vi "Actividad 1-Tanque.vi"() -> ()   [LabVIEW 2018]
panel:
  in  "stop":bool
  in  "Decremento":bool
  in  "Incremento":bool
  out "Tank":dbl(slide) scale=0.0..10.0
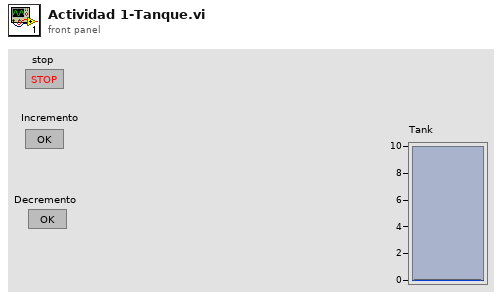
[diagram p1: front panel]
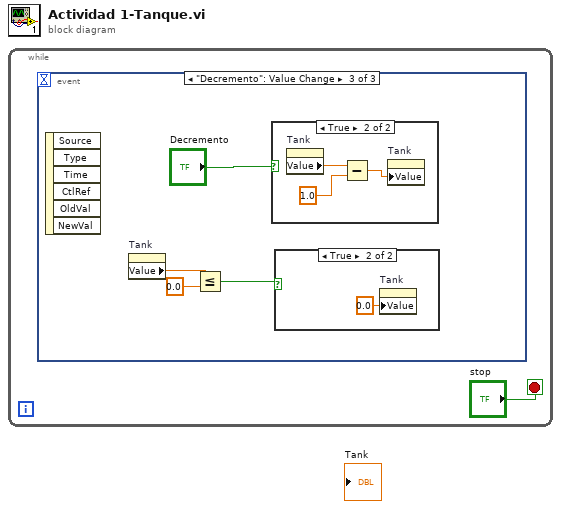
[diagram p0: block diagram]
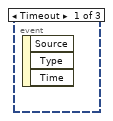
[diagram p2: hidden frame]
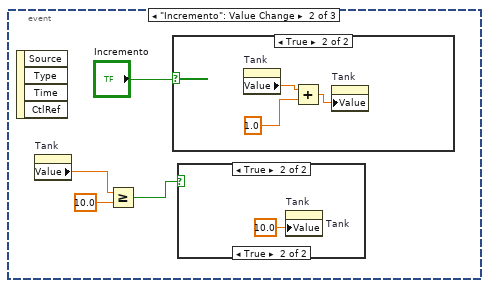
[diagram p3: hidden frame]
diagram:
  n1 = while {
    stop <- "stop" stop-if-true
    n2 = event shown="[2] \"Decremento\": Value Change" {
      selector: _ -> [_ _ _]
      dyn-events: _ -> [_ _ _]
      timeout: _ -> [_ _ _]
      event Timeout {
        n3 = event-data() -> ()  [unwired: 1 in, 3 out]
      }
      event "Incremento": Value Change {
        n4 = event-data() -> ()  [unwired: 1 in, 4 out]
        n5 = property on="Tank" class="Slide (strict)"() -> ("Value"=w3:dbl)  [unwired: 2 in, 2 out]
        n6 = Greater Or Equal?(x=w3, y=10.0) -> (x >= y?=w2:bool)
        n7 = case shown="True" "Incremento" {
          frame False {
          }
          frame True {
            n8 = property on="Tank" class="Slide (strict)"() -> ("Value"=w9:dbl)  [unwired: 2 in, 2 out]
            n9 = Add(x=w9, y=1.0) -> (x+y=w8:dbl)
            n10 = property on="Tank" class="Slide (strict)"("Value"=w8) -> ()  [unwired: 2 in, 2 out]
          }
        }
        n11 = case shown="True" {
          selector: _ -> [_ _]
          frame False {
          }
          frame True {
            n12 = property on="Tank" class="Slide (strict)"("Value"=10.0 ("Tank")) -> ()  [unwired: 2 in, 2 out]
          }
        }
        n13 = case shown="True" w2 {
          frame False {
          }
          frame True {
            n14 = property on="Tank" class="Slide (strict)"("Value"=10.0 ("Tank")) -> ()  [unwired: 2 in, 2 out]
          }
        }
      }
      event "Decremento": Value Change {
        n15 = event-data() -> ()  [unwired: 1 in, 6 out]
        n16 = property on="Tank" class="Slide (strict)"() -> ("Value"=w12:dbl)  [unwired: 2 in, 2 out]
        n17 = Less Or Equal?(x=w12, y=0.0) -> (x <= y?=w11:bool)
        n18 = case shown="True" "Decremento" {
          frame False {
          }
          frame True {
            n19 = property on="Tank" class="Slide (strict)"() -> ("Value"=w17:dbl)  [unwired: 2 in, 2 out]
            n20 = Subtract(x=w17, y=1.0) -> (x-y=w16:dbl)
            n21 = property on="Tank" class="Slide (strict)"("Value"=w16) -> ()  [unwired: 2 in, 2 out]
          }
        }
        n22 = case shown="True" w11 {
          frame False {
          }
          frame True {
            n23 = property on="Tank" class="Slide (strict)"("Value"=0.0 ("Tank")) -> ()  [unwired: 2 in, 2 out]
          }
        }
      }
    }
  }
